vi "Decimate File.vi"(7 "Output file path (dialog if empty) 2":path, 8 "error in (no error)":errorcluster, 10 "Decimate by":i32=16, 11 "file path (dialog if empty)":path) -> (0 "error out":errorcluster, 3 "new file path (Not A Path if cancelled)":path)   [LabVIEW 2015]
uses:
  <vilib>/Analysis/2dsp.llb/Decimate (single shot, DBL).vi
  <vilib>/Analysis/NI_AALPro.lvlib
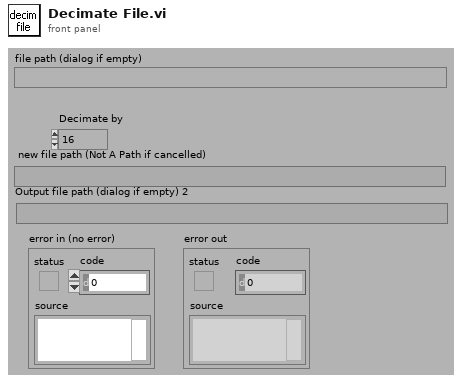
[diagram p1: front panel]
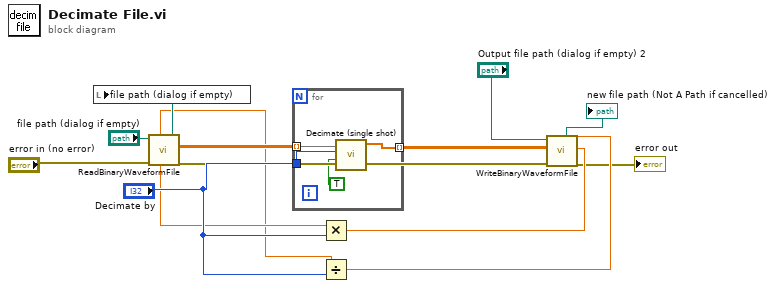
[diagram p0: block diagram]
diagram:
  n1 = call "ReadBinaryWaveformFile.vi"("error in (no error)"="error in (no error)", "file path (dialog if empty)"="file path (dialog if empty)") -> ("error out"=w1:errorcluster, "2D array"=w13:sgl[][], "new file path (Not A Path if cancelled)"=w10:path, "Time base"=w7:dbl, "Delay, points"=w5:dbl)  [unwired: 2 in, 3 out]
  n2 = local write "file path (dialog if empty)"(w10) -> ()
  n3 = for {
    tunnel: w13 -> [w18] mode=indexing
    tunnel: "Decimate by" -> [w16]
    tunnel: [w15] -> w12 mode=indexing
    n4 = call-poly <vilib>:"Decimate (single shot).vi"("averaging"=TRUE, "decimating factor"=w16, "X"=w18) -> ("Decimated Array"=w15:dbl[])  [unwired: 7 in, 1 out]
  }
  n5 = Multiply(x=w7, y="Decimate by") -> (x*y=w6:dbl)
  n6 = Divide(x=w5, y="Decimate by") -> (x/y=w4:dbl)
  n7 = call "WriteBinaryWaveformFile.vi"("Time base"=w6, "Delay, points"=w4, "error in (no error)"=w1, "2D array"=w12, "file path (dialog if empty)"="Output file path (dialog if empty) 2") -> ("error out"=→"error out":errorcluster, "new file path (Not A Path if cancelled)"=→"new file path (Not A Path if cancelled)":path)  [unwired: 5 in]
